vi "Create Serial Input Channel I2C IO x2.vi"() -> (4 "serial input channel i2c io x2":T2)   [LabVIEW 2020, in "GettingStarted_Common_148X_FPGA.lvlib"]
uses:
  GettingStarted_Common_148X_FPGA.lvlib
  Types/I2C IO.ctl
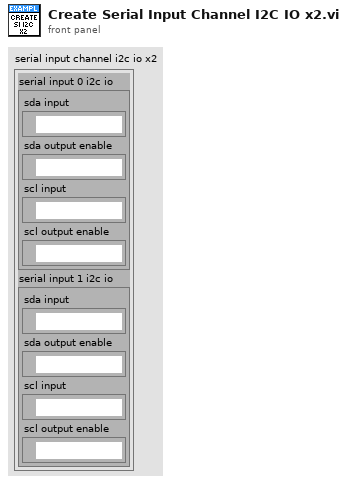
[diagram p1: front panel]
types:
  T1 = typedef "GettingStarted_Common_148X_FPGA.lvlib/I2C IO.ctl" = cluster{"sda input":refnum<k21>, "sda output enable":refnum<k21>, "scl input":refnum<k21>, "scl output enable":refnum<k21>}
  T2 = cluster{"serial input 0 i2c io":T1, "serial input 1 i2c io":T1}
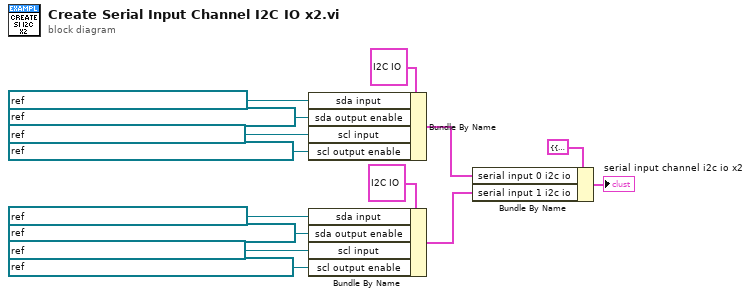
[diagram p0: block diagram]
diagram:
  n1 = Bundle By Name(cluster=T1 {"sda input"="IO Socket\\SI 0 Deserializer I2C SDA Input", "sda output enable"="IO Socket\\SI 0 Deserializer I2C SDA Output Enable", "scl input"="IO Socket\\SI 0 Deserializer I2C SCL Input", "scl output enable"="IO Socket\\SI 0 Deserializer I2C SCL Output Enable"}, "sda input"=refnum<k21> "IO Socket\\SI 0 Deserializer I2C SDA Input", "sda output enable"=refnum<k21> "IO Socket\\SI 0 Deserializer I2C SDA Output Enable", "scl input"=refnum<k21> "IO Socket\\SI 0 Deserializer I2C SCL Input", "scl output enable"=refnum<k21> "IO Socket\\SI 0 Deserializer I2C SCL Output Enable") -> (w13:T1)
  n2 = Bundle By Name(cluster=T1 {"sda input"="IO Socket\\SI 0 Deserializer I2C SDA Input", "sda output enable"="IO Socket\\SI 0 Deserializer I2C SDA Output Enable", "scl input"="IO Socket\\SI 0 Deserializer I2C SCL Input", "scl output enable"="IO Socket\\SI 0 Deserializer I2C SCL Output Enable"}, "sda input"=refnum<k21> "IO Socket\\SI 1 Deserializer I2C SDA Input", "sda output enable"=refnum<k21> "IO Socket\\SI 1 Deserializer I2C SDA Output Enable", "scl input"=refnum<k21> "IO Socket\\SI 1 Deserializer I2C SCL Input", "scl output enable"=refnum<k21> "IO Socket\\SI 1 Deserializer I2C SCL Output Enable") -> (w14:T1)
  n3 = Bundle By Name(cluster=T2 {"serial input 0 i2c io"={"sda input"="", "sda output enable"="", "scl input"="", "scl output enable"=""}, "serial input 1 i2c io"={"sda input"="", "sda output enable"="", "scl input"="", "scl output enable"=""}} ("serial input channel i2c io x2"), "serial input 0 i2c io"=w13, "serial input 1 i2c io"=w14) -> (→"serial input channel i2c io x2":T2)
